vi "Actor Core.vi"(8 "error in":errorcluster, 11 "Room Service Monitor UI in":refnum<class "Room Service Monitor UI.lvclass">) -> (0 "error out":errorcluster, 3 "Actor out":refnum<class "Actor.lvclass">)   [LabVIEW 2023, in "Room Service Monitor UI.lvlib" / "Room Service Monitor UI.lvclass"]
doc: "(<B>Filename</B>: Actor Framework.lvlib:Actor.lvclass:Actor Core.vi)\n\nReceives messages to the actor, reacts to them, and initiates any error handling that may shut the actor down.\n\nDescendant classes may override this VI to append parallel tasks for the actor to complete while it handles messages. Overrides use the Call Parent Class Method node."
uses:
  Room Service Monitor UI.lvclass
  C:/Users/bhaghyaraj/Trainings/NI Actor Framework/SDLC/UI Base/UI Base/UI Base.lvclass
  C:/Program Files/National Instruments/LabVIEW 2023/vi.lib/ActorFramework/Actor/Actor.lvclass
  <vilib>/ActorFramework/Actor/Actor.lvclass
  Room Service Monitor UI.lvclass/Room Service Monitor UI.ctl
  <vilib>/ActorFramework/Actor/Actor.lvclass/Actor.ctl
  <vilib>/ActorFramework/Message Enqueuer/Message Enqueuer.lvclass/Message Enqueuer.ctl
  <vilib>/ActorFramework/Message Enqueuer/Init from Existing Queue.vi
  <vilib>/ActorFramework/Message Enqueuer/Enqueue.vi
  Room Service Monitor UI Messages/Initialize UI Msg/Initialize UI Msg.lvclass
  C:/Program Files/National Instruments/LabVIEW 2023/vi.lib/ActorFramework/Message/Message.lvclass
  <vilib>/ActorFramework/Stop Msg/Stop Msg.lvclass
  <vilib>/ActorFramework/Message Priority Queue/Priority Enqueue.vi
  <vilib>/ActorFramework/Message Enqueuer/Message Enqueuer.lvclass
  UI Base/UI Base/UI Base.lvclass
  Room Service Monitor UI Messages/Complete Service Msg/Complete Service Msg.lvclass
panel:
  in  "Complete":bool
  out "Service Description":string
  out "Allocated Staff":string
  out "Title":string
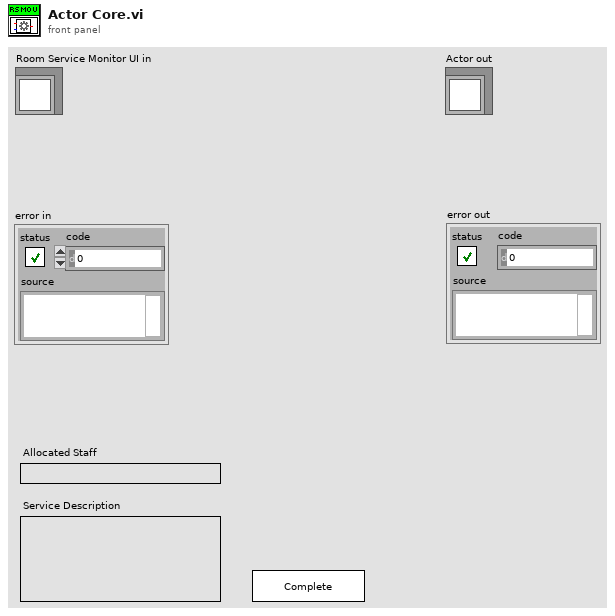
[diagram p1: front panel]
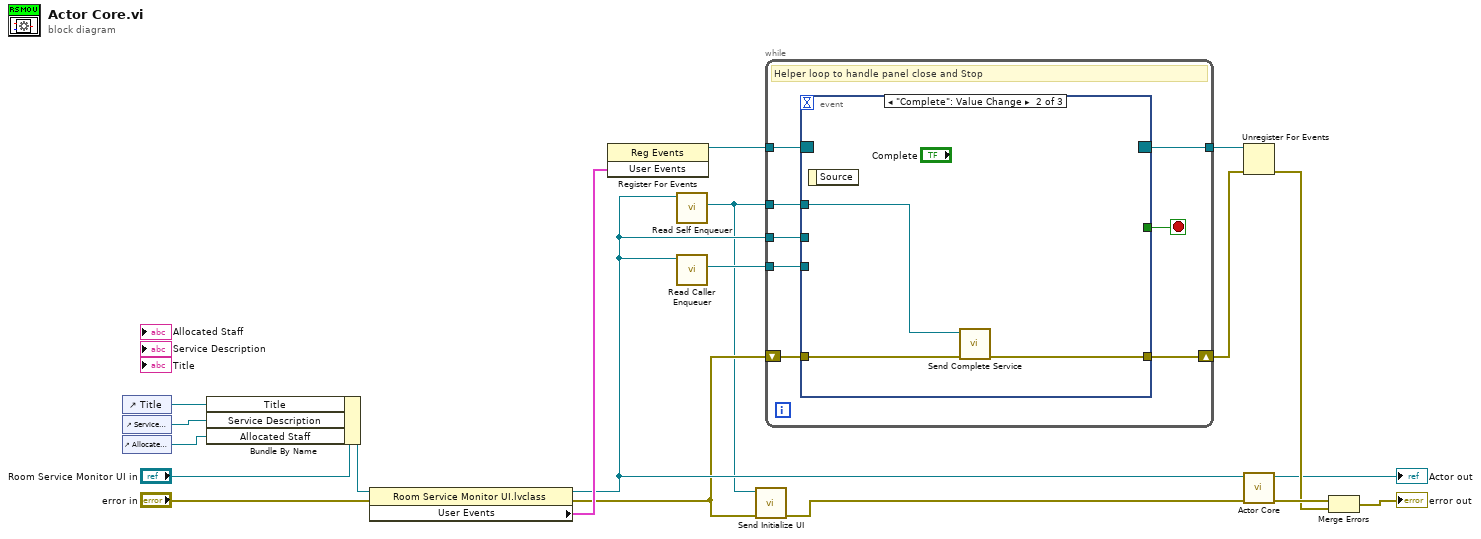
[diagram p0: block diagram]
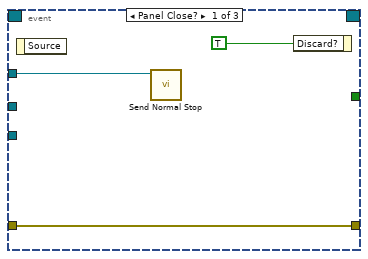
[diagram p2: hidden frame]
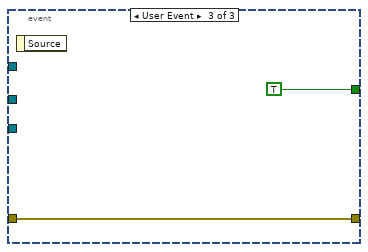
[diagram p3: hidden frame]
diagram:
  n1 = control-ref of="Title"() -> (w5:refnum<vi>)
  n2 = control-ref of="Service Description"() -> (w4:refnum<vi>)
  n3 = control-ref of="Allocated Staff"() -> (w3:refnum<vi>)
  n4 = Bundle By Name(cluster="Room Service Monitor UI in", "Title"=w5, "Service Description"=w4, "Allocated Staff"=w3) -> (w6:refnum<class "Room Service Monitor UI.lvclass">)
  n5 = property class="Room Service Monitor UI.lvclass"(reference=w6, error in="error in") -> (reference out=w13:refnum<class "Room Service Monitor UI.lvclass">, error out=w12:errorcluster, "User Events"=w16:cluster{"Stop":refnum<user-event>})
  n6 = register-events(w16) -> (reference out=w17:refnum<event-registration>)  [unwired: 2 in, 1 out]
  n7 = call <vilib>:"Read Self Enqueuer.vi"("Actor"=w13) -> ("Self Enqueuer"=w1:refnum<class "Message Enqueuer.lvclass">)  [unwired: 10 in]
  n8 = call <vilib>:"Read Caller Enqueuer.vi"("Actor"=w13) -> ("Caller Enqueuer"=w14:refnum<class "Message Enqueuer.lvclass">)  [unwired: 10 in]
  n9 = call "Send Initialize UI.vi"("error in (no error)"=w12, "Message Enqueuer"=w1) -> ("error out"=w2:errorcluster)  [unwired: 8 in, 1 out]
  n10 = while {
    tunnel: w1 -> [w27]
    tunnel: w17 -> [w26]
    tunnel: [w24] -> w18
    tunnel: w14 -> [w23]
    tunnel: w13 -> [w22]
    shift-right: [w20] -> w11
    shift-left: w12 -> [w21]
    stop <- w25 stop-if-true
    # "Helper loop to handle panel close and Stop"
    n11 = event shown="[1] \"Complete\": Value Change" {
      selector: w26 -> [_ _ _]
      dyn-events: [_ _ _] -> w24
      timeout: _ -> [_ _ _]
      tunnel: w27 -> [w29 w31 _]
      tunnel: [_ _ TRUE] -> w25
      tunnel: w23 -> [_ _ _]
      tunnel: w22 -> [_ _ _]
      tunnel: w21 -> [w28 w33 w34]
      tunnel: [w28 w32 w34] -> w20
      event Panel Close? {
        n12 = event-data() -> ()  [unwired: 1 in, 1 out]
        n13 = call <vilib>:"Send Normal Stop.vi"("Message Enqueuer"=w29) -> ()  [unwired: 10 in, 1 out]
        n14 = event-data("Discard?"=TRUE) -> ()  [unwired: 1 in, 1 out]
      }
      event "Complete": Value Change {
        n15 = event-data() -> ()  [unwired: 1 in, 1 out]
        n16 = call "Send Complete Service.vi"("error in (no error)"=w33, "Message Enqueuer"=w31) -> ("error out"=w32:errorcluster)  [unwired: 8 in, 1 out]
      }
      event User Event {
        n17 = event-data() -> ()  [unwired: 1 in, 1 out]
      }
    }
  }
  n18 = Unregister For Events(event registration refnum=w18, error in=w11) -> (error out=w15:errorcluster)
  n19 = call-parent "Actor Core.vi"("error in"=w2, "Actor in"=w13) -> ("error out"=w19:errorcluster, "Actor out"=→"Actor out":refnum<class "Actor.lvclass">)  [unwired: 8 in]
  n20 = Merge Errors(w19, w15) -> (→"error out":errorcluster)
